vi "RH_PPMU_Disconnect.vi"(8 "error in":errorcluster, 10 "channel list":string, 11 "PPMU Session In":refnum<k15>) -> (0 "error out":errorcluster, 3 "PPMU Session Out":refnum<k15>)   [LabVIEW 2023, in "ResourceHandling.lvlib"]
doc: "Disconnect the PPMU channels"
uses:
  ResourceHandling.lvlib
  <instrlib>/niDigital/niDigital.llb/niDigital Selected Function.ctl
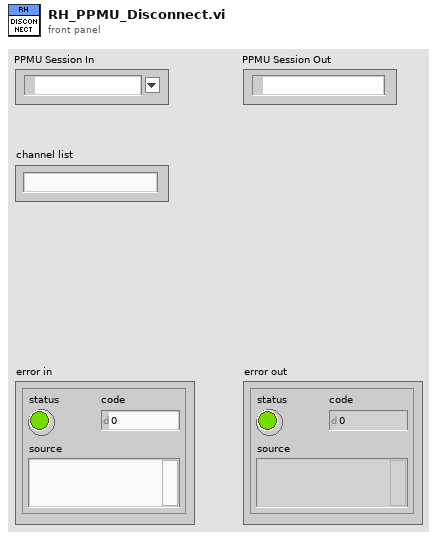
[diagram p1: front panel]
types:
  T1 = typedef "niDigital Selected Function.ctl" = i32
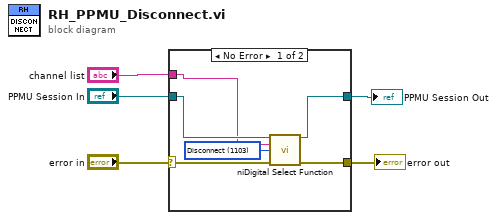
[diagram p0: block diagram]
diagram:
  n1 = case shown="No Error" "error in" {
    selector: "error in" -> [w11 w12]
    tunnel: "PPMU Session In" -> [w9 w13]
    tunnel: "channel list" -> [w7 _]
    tunnel: [w10 w12] -> w3
    tunnel: [w8 w13] -> w4
    frame No Error {
      w6 = T1 1103 items=["Digital"=1100, "PPMU"=1101, "Off"=1102, "Disconnect"=1103, "RIO"=1104] ("function")
      n2 = call <instrlib>:"niDigital Select Function.vi"("instrument handle"=w9, "channel list"=w7, "function"=w6, "error in"=w11) -> ("instrument handle out"=w8:refnum<k15>, "error out"=w10:errorcluster)  [unwired: 10 in]
    }
    frame Error {
    }
  }
  "error out" <- w3
  "PPMU Session Out" <- w4
